vi "Main.vi"() -> ()   [LabVIEW 2015, in "Display.lvlib"]
doc: "This template is based off of the Queued Message Handler design pattern and the Queued Message Handler project template that ships with LabVIEW.\n\nThe main difference is that the queue is private to this module and communication between modules is performed via Broadcast and Request events.\n\nRequest events are wrapped in public API methods and are handled in the Event Handling Loop (EHL) of this VI. Any module can register for Broadcast events sent by this module. The EHL generates messages based on user interface actions.\n\nThe Message Handling Loop (MHL) processes messages generated by the EHL, or by other messages. The messages are string values, so new messages can be added easily to the Message Cases case structure in the MHL. Each message cluster can also provide an optional value for Message Data, which is a variant that can be converted to whatever message-specific data is required.\n_____\nBased on Delacor QMH Project Template 4.2.1.64."
uses:
  Display.lvlib
  <vilib>/Delacor/Delacor QMH/Libraries/Module Admin_class/Delacor_lib_QMH_Module Admin.lvclass
  Module Data--cluster.ctl
  <vilib>/Delacor/Delacor QMH/Libraries/Message Queue_class/Delacor_lib_QMH_Message Queue.lvclass/Delacor_lib_QMH_Message Queue.ctl
  Stop Argument--cluster.ctl
  <vilib>/Delacor/Delacor QMH/Libraries/Module Admin_class/Delacor_lib_QMH_Module Admin.lvclass/Delacor_lib_QMH_Module Admin.ctl
  Update Display Argument--cluster.ctl
  <vilib>/Utility/miscctls.llb/LVPointTypeDef.ctl
  <vilib>/Delacor/Delacor QMH/Libraries/Message Queue_class/Delacor_lib_QMH_Enqueue Message (Single).vi
  <vilib>/Delacor/Delacor QMH/Libraries/Module Admin_class/Delacor_lib_QMH_Get External Launch.vi
  <vilib>/Utility/error.llb/Error Cluster From Error Code.vi
  <vilib>/ErrorRing/Error Ring.xnode
  <vilib>/Delacor/Delacor QMH/Libraries/Message Queue_class/Delacor_lib_QMH_Message Queue.lvclass
panel:
  out "Display":string
  in  "Simulate MHL Error":bool
  in  "Simulate EHL Error":bool
  out "error out":errorcluster
  in  "Module Admin":refnum<class "Delacor_lib_QMH_Module Admin.lvclass">
  out "Status":string
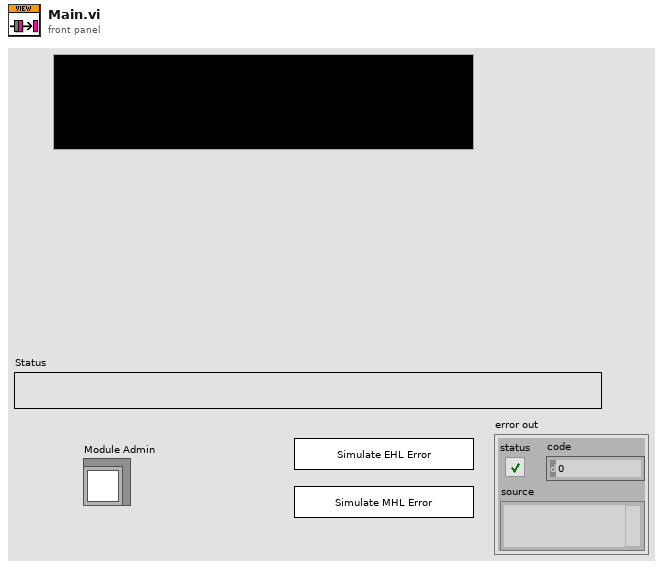
[diagram p1: front panel]
types:
  T1 = typedef "Display.lvlib/Request Events--cluster.ctl" = cluster{"Stop Module":refnum<user-event>, "Show Panel":refnum<user-event>, "Hide Panel":refnum<user-event>, "Get Module Execution Status":refnum<user-event>, "Show Diagram":refnum<user-event>, "Update Display":refnum<user-event>}
  T2 = typedef "Display.lvlib/Module Data--cluster.ctl" = cluster{"Status":string, "Balance (for indication only)":u32}
  T3 = enum32{"invalid lock state", "Not Locked", "Locked (No Password)", "Password-protected"}
  T4 = typedef "Display.lvlib/Stop Argument--cluster.ctl" = cluster{"Origin":string, "Exit via Stop Module Req?":bool, "Wait for Module to stop?":bool}
  T5 = typedef "Display.lvlib/Update Display Argument--cluster.ctl" = cluster{"Message to display":string, "Balance":u32}
  T6 = typedef "LVPointTypeDef.ctl" = cluster{"Horizontal":i16, "Vertical":i16}
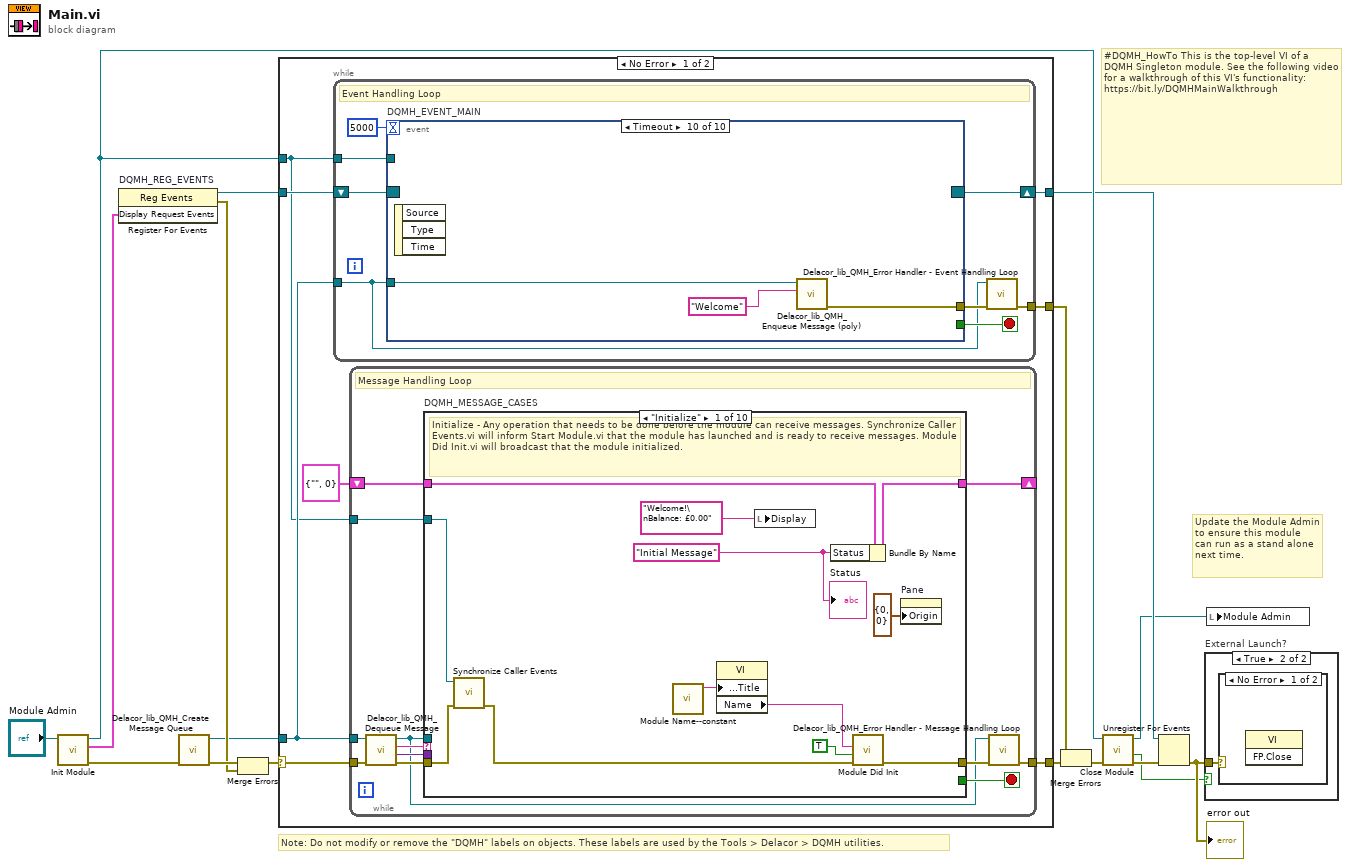
[diagram p0: block diagram]
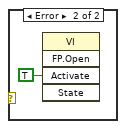
[diagram p3: hidden frame]
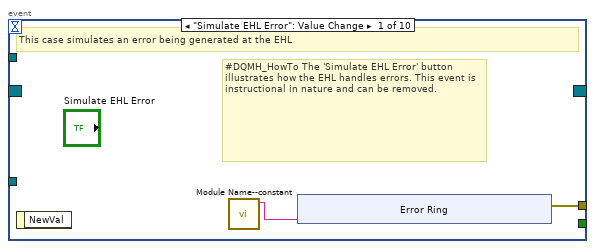
[diagram p4: hidden frame]
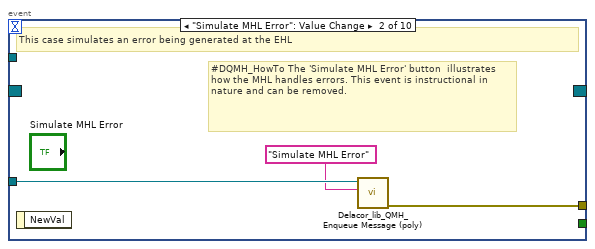
[diagram p5: hidden frame]
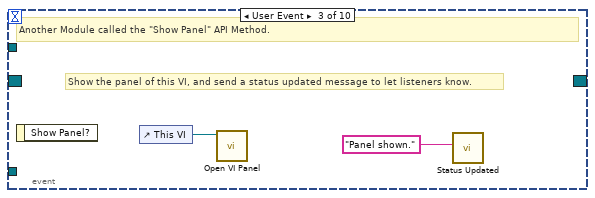
[diagram p6: hidden frame]
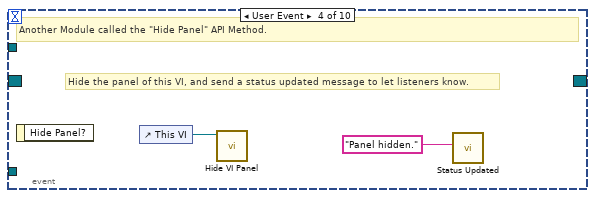
[diagram p7: hidden frame]
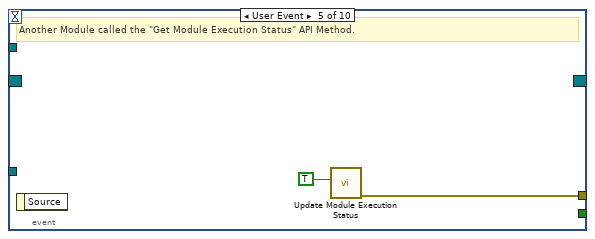
[diagram p8: hidden frame]
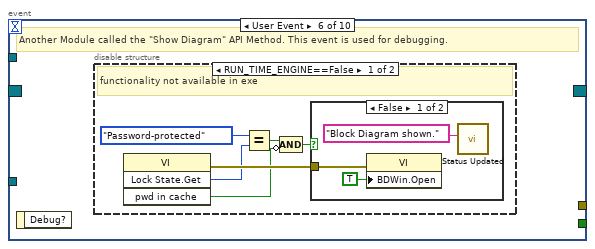
[diagram p9: hidden frame]
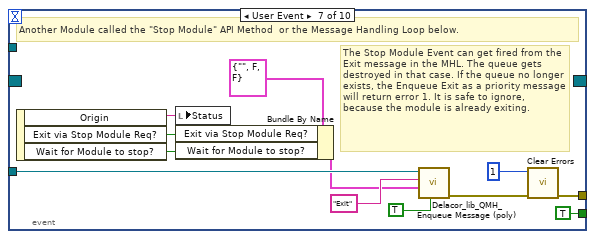
[diagram p12: hidden frame]
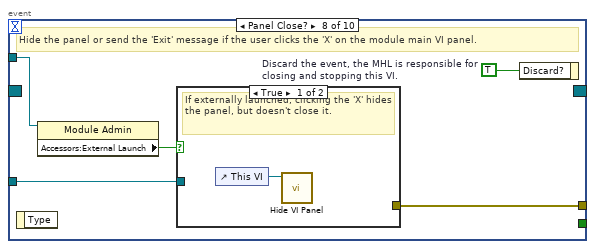
[diagram p13: hidden frame]
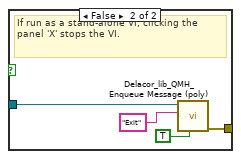
[diagram p14: hidden frame]
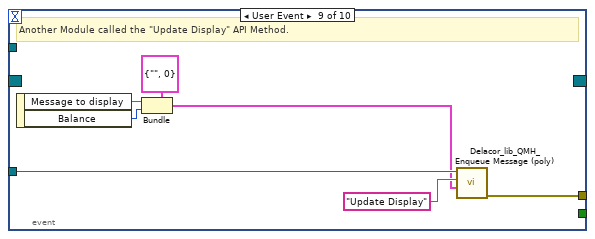
[diagram p15: hidden frame]
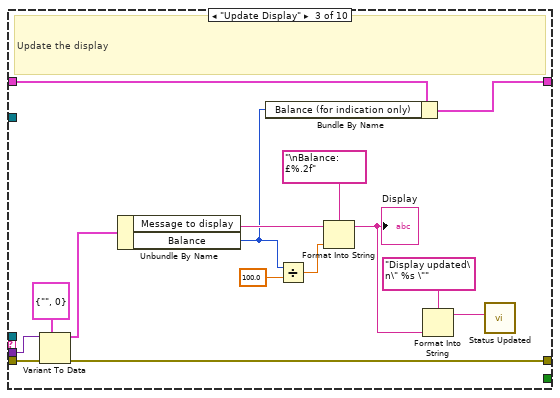
[diagram p17: hidden frame]
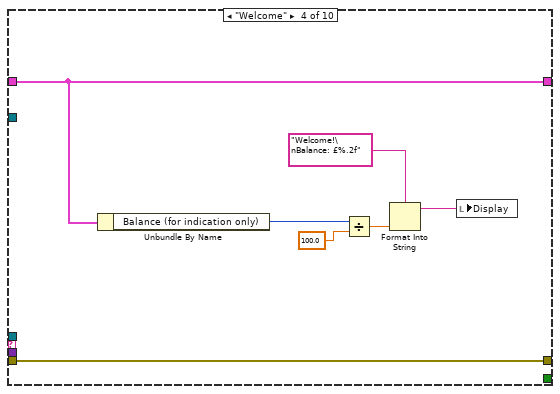
[diagram p18: hidden frame]
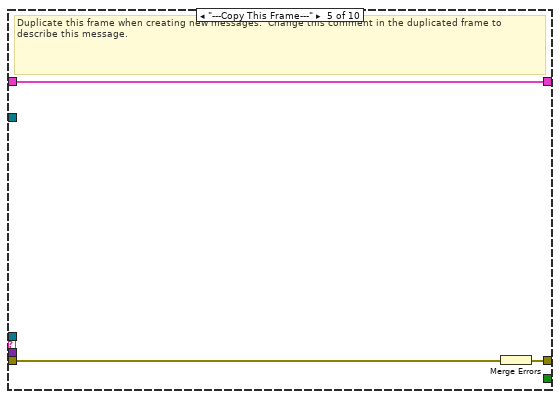
[diagram p19: hidden frame]
diagram:
  # "#DQMH_HowTo This is the top-level VI of a DQMH Singleton module. See the following video for a walkthrough of this VI's functionality: https://bit.ly/DQMHMainWalkthrough"
  # "Note: Do not modify or remove the \"DQMH\" labels on objects. These labels are used by the Tools > Delacor > DQMH utilities."
  # "Update the Module Admin to ensure this module can run as a stand alone next time."
  n1 = call "Init Module.vi"("Singleton Module Admin in"="Module Admin") -> ("error out"=w16:errorcluster, "Display Request Events"=w5:T1, "Singleton Module Admin out"=w8:refnum<class "Delacor_lib_QMH_Module Admin.lvclass">)  [unwired: 8 in]
  n2 = register-events "DQMH_REG_EVENTS"(w5) -> (reference out=w6:refnum<event-registration>, error out=w9:errorcluster)  [unwired: 2 in]
  n3 = call <vilib>:"Delacor_lib_QMH_Create Message Queue.vi"("error in (no error)"=w16) -> ("error out"=w11:errorcluster, "Message Queue"=w4:refnum<class "Delacor_lib_QMH_Message Queue.lvclass">)  [unwired: 9 in]
  n4 = Merge Errors(w11, w9) -> (w10:errorcluster)
  n5 = case shown="No Error" w10 {
    selector: w10 -> [w23 w210]
    tunnel: [w25 w210] -> w17
    tunnel: [w22 w207] -> w7
    tunnel: w6 -> [w20 w207]
    tunnel: w4 -> [w19 _]
    tunnel: [w24 _] -> w14
    tunnel: w8 -> [w18 w203]
    frame No Error {
      n6 = while {
        tunnel: w19 -> [w27]
        shift-right: [w30] -> w22
        shift-left: w20 -> [w31]
        tunnel: [w32] -> w24
        tunnel: w18 -> [w28]
        stop <- w29 stop-if-true
        # "Event Handling Loop"
        n7 = event "DQMH_EVENT_MAIN" shown="[9] Timeout" {
          selector: w31 -> [_ _ _ _ _ _ _ _ _ _]
          dyn-events: [_ _ _ _ _ _ _ _ _ _] -> w30
          timeout: 5000 -> [_ _ _ _ _ _ _ _ _ _]
          tunnel: [_ _ _ _ _ _ TRUE ("Discard?") _ _ _] -> w29
          tunnel: w27 -> [_ w44 _ _ _ _ w68 w75 w89 w90]
          tunnel: [w35 w45 _ _ w51 _ w71 w77 w84 w91] -> w33
          tunnel: w28 -> [_ _ _ _ _ _ _ w74 _ _]
          event "Simulate EHL Error": Value Change {
            # "#DQMH_HowTo The 'Simulate EHL Error' button  illustrates how the EHL handles errors. This event is instructional in nature and can be removed."
            # "This case simulates an error being generated at the EHL"
            n8 = event-data() -> ()  [unwired: 1 in, 1 out]
            n9 = call "Module Name--constant.vi"() -> ("Module Name"=w34:string)  [unwired: 11 in]
            n10 = xnode "Error Ring"("parameter 0"=w34) -> ("error out"=w35:errorcluster)
          }
          event "Simulate MHL Error": Value Change {
            # "#DQMH_HowTo The 'Simulate MHL Error' button  illustrates how the MHL handles errors. This event is instructional in nature and can be removed."
            # "This case simulates an error being generated at the EHL"
            n11 = event-data() -> ()  [unwired: 1 in, 1 out]
            n12 = call-poly <vilib>:"Delacor_lib_QMH_Enqueue Message (poly).vi"("Message"="Simulate MHL Error", "Message Queue in"=w44) -> ("error out"=w45:errorcluster)  [unwired: 8 in, 1 out]
          }
          event User Event {
            # "Show the panel of this VI, and send a status updated message to let listeners know."
            # "Another Module called the \"Show Panel\" API Method."
            n13 = event-data() -> ()  [unwired: 1 in, 1 out]
            n14 = control-ref of="This VI"() -> (w47:refnum<vi>)
            n15 = call "Open VI Panel.vi"("VI"=w47) -> ()  [unwired: 10 in, 1 out]
            n16 = call "Status Updated.vi"("Status"="Panel shown." ("format string")) -> ()  [unwired: 10 in, 1 out]
          }
          event User Event {
            # "Hide the panel of this VI, and send a status updated message to let listeners know."
            # "Another Module called the \"Hide Panel\" API Method."
            n17 = event-data() -> ()  [unwired: 1 in, 1 out]
            n18 = control-ref of="This VI"() -> (w49:refnum<vi>)
            n19 = call "Hide VI Panel.vi"("VI"=w49) -> ()  [unwired: 10 in, 1 out]
            n20 = call "Status Updated.vi"("Status"="Panel hidden." ("format string")) -> ()  [unwired: 10 in, 1 out]
          }
          event User Event {
            # "Another Module called the \"Get Module Execution Status\" API Method."
            n21 = event-data() -> ()  [unwired: 1 in, 1 out]
            n22 = call "Update Module Execution Status.vi"("Running?"=TRUE) -> ("error out"=w51:errorcluster)  [unwired: 10 in]
          }
          event User Event {
            # "Another Module called the \"Show Diagram\" API Method. This event is used for debugging."
            n23 = event-data() -> ()  [unwired: 1 in, 1 out]
            n24 = disable-structure shown="RUN_TIME_ENGINE==False" {
              frame condition #0 (active) {
                # "functionality not available in exe"
                n25 = invoke class="VI" method="Lock State.Get"() -> (error out=w57:errorcluster, "Get Lock State"=w56:T3, "pwd in cache"=w53:bool)  [unwired: 4 in, 1 out]
                n26 = Equal?(x=T3."Password-protected", y=w56) -> (x = y?=w54:bool)
                n27 = Compound Arithmetic op=AND(w54, invert w53) -> (w52:bool)
                n28 = case shown="False" w52 {
                  tunnel: w57 -> [w60 _]
                  frame False {
                    n29 = property class="VI"(error in=w60, "BDWin.Open"=TRUE ("Block Diagram Window:Open")) -> ()  [unwired: 1 in, 2 out]
                    n30 = call "Status Updated.vi"("Status"="Block Diagram shown." ("format string")) -> ()  [unwired: 10 in, 1 out]
                  }
                  frame True {
                    # "Password-protected VI, and the password is not in the cache. Do not show the diagram."
                  }
                }
              }
              frame condition #1 {
              }
            }
          }
          event User Event {
            # "The Stop Module Event can get fired from the Exit message in the MHL. The queue gets destroyed in that case. If the queue no longer exists, the Enqueue Exit as a priority message will return error 1. It is safe to ignore, because the module is already exiting."
            # "Another Module called the \"Stop Module\" API Method  or the Message Handling Loop below."
            n31 = event-data() -> ("Origin"=w67:string, "Exit via Stop Module Req?"=w63:bool, "Wait for Module to stop?"=w62:bool)  [unwired: 1 in]
            n32 = local write "Status"(w67) -> ()
            n33 = Bundle By Name(cluster=T4 {"Origin"="", "Exit via Stop Module Req?"=FALSE, "Wait for Module to stop?"=FALSE} ("Stop Argument"), "Exit via Stop Module Req?"=w63, "Wait for Module to stop?"=w62) -> (w61:T4)
            n34 = call-poly <vilib>:"Delacor_lib_QMH_Enqueue Message (poly).vi"("Priority Message? (F)"=TRUE, "Message Data"=w61, "Message"="Exit", "Message Queue in"=w68) -> ("error out"=w72:errorcluster)  [unwired: 6 in, 1 out]
            n35 = call <vilib>:"Clear Errors.vi"("error in (no error)"=w72, "specific error code to clear (0: all)"=1) -> ("error out"=w71:errorcluster)  [unwired: 4 in, 1 out]
          }
          event Panel Close? {
            w76 = TRUE  # Discard the event, the MHL is responsible for closing and stopping this VI.
            # "Hide the panel or send the 'Exit' message if the user clicks the 'X' on the module main VI panel."
            n36 = event-data() -> ()  [unwired: 1 in, 1 out]
            n37 = property class="Module Admin"(reference=w74) -> ("Accessors:External Launch"=w73:bool)  [unwired: 1 in, 2 out]
            n38 = case shown="True" w73 {
              tunnel: w75 -> [_ w81]
              tunnel: [_ w82] -> w77
              frame True {
                # "If externally launched, clicking the 'X' hides the panel, but doesn't close it."
                n39 = control-ref of="This VI"() -> (w78:refnum<vi>)
                n40 = call "Hide VI Panel.vi"("VI"=w78) -> ()  [unwired: 10 in, 1 out]
              }
              frame False {
                # "If run as a stand-alone VI, clicking the panel 'X' stops the VI."
                n41 = call-poly <vilib>:"Delacor_lib_QMH_Enqueue Message (poly).vi"("Priority Message? (F)"=TRUE, "Message"="Exit", "Message Queue in"=w81) -> ("error out"=w82:errorcluster)  [unwired: 7 in, 1 out]
              }
            }
            n42 = event-data("Discard?"=w76) -> ()  [unwired: 1 in, 1 out]
          }
          event User Event {
            # "Another Module called the \"Update Display\" API Method."
            n43 = event-data() -> ("Message to display"=w85:string, "Balance"=w83:u32)  [unwired: 1 in]
            n44 = Bundle(cluster=T5 {"Message to display"="", "Balance"=0} ("Update Display Argument"), "Message to display"=w85, "Balance"=w83) -> (w86:T5)
            n45 = call-poly <vilib>:"Delacor_lib_QMH_Enqueue Message (poly).vi"("Message Data"=w86, "Message"="Update Display", "Message Queue in"=w89) -> ("error out"=w84:errorcluster)  [unwired: 7 in, 1 out]
          }
          event Timeout {
            n46 = event-data() -> ()  [unwired: 1 in, 3 out]
            n47 = call-poly <vilib>:"Delacor_lib_QMH_Enqueue Message (poly).vi"("Message"="Welcome", "Message Queue in"=w90) -> ("error out"=w91:errorcluster)  [unwired: 8 in, 1 out]
          }
        }
        n48 = call-dynamic "Delacor_lib_QMH_Error Handler - Event Handling Loop.vi"("error in (no error)"=w33, "Message Queue in"=w27) -> ("dup error in"=w32:errorcluster)  [unwired: 8 in, 1 out]
      }
      n49 = while {
        tunnel: w19 -> [w95]
        shift-right: [w99] -> _
        shift-left: T2 {"Status"="", "Balance (for indication only)"=0} ("Data Cluster") -> [w100]
        tunnel: w23 -> [w103]
        tunnel: [w101] -> w25
        tunnel: w18 -> [w93]
        stop <- w98 stop-if-true
        # "Message Handling Loop"
        n50 = call-dynamic "Delacor_lib_QMH_Dequeue Message.vi"("error in (no error)"=w103, "Message Queue in"=w95) -> ("error out"=w102:errorcluster, "Message Data"=w96:variant, "Message"=w97:string, "Message Queue out"=w94:refnum<class "Delacor_lib_QMH_Message Queue.lvclass">)  [unwired: 6 in]
        n51 = case "DQMH_MESSAGE_CASES" shown="\"Initialize\"" w97 {
          selector: w97 -> [_ _ _ _ _ _ _ _ _ w190]
          tunnel: w94 -> [_ _ _ _ _ _ _ w160 w182 _]
          tunnel: w102 -> [w116 w118 w133 w140 w143 w145 w150 w167 w188 w192]
          tunnel: [w114 w118 w132 w140 w142 w145 w149 w163 w185 w193] -> w104
          tunnel: w100 -> [w111 w117 w124 w135 w141 w144 w147 w162 w181 w191]
          tunnel: [w110 w117 w122 w135 w141 w144 w147 w162 w181 w191] -> w99
          tunnel: [_ _ _ _ _ _ _ _ w180 _] -> w98
          tunnel: w96 -> [_ _ w131 _ _ _ _ w161 w179 _]
          tunnel: w93 -> [w112 _ _ _ _ _ _ w159 w174 _]
          frame "Initialize" {
            w107 = "Initial Message" ("Initial Message")
            # "Initialize - Any operation that needs to be done before the module can receive messages. Synchronize Caller Events.vi will inform Start Module.vi that the module has launched and is ready to receive messages. Module Did Init.vi will broadcast that the module initialized."
            n52 = call "Synchronize Caller Events.vi"("error in (no error)"=w116, "Singleton Module Admin in"=w112) -> ("error out"=w115:errorcluster)  [unwired: 8 in, 1 out]
            n53 = call "Module Name--constant.vi"() -> ("Module Name"=w113:string)  [unwired: 11 in]
            n54 = property class="VI"("Front Panel.Title"=w113) -> ("Name"=w105:string)  [unwired: 2 in, 2 out]
            n55 = local write "Display"("Welcome!\nBalance: £0.00" ("Display")) -> ()
            n56 = Bundle By Name(cluster=w111, "Status"=w107) -> (w110:T2)
            n57 = call "Module Did Init.vi"("error in (no error)"=w115, "Initialized?"=TRUE, "Origin"=w105) -> ("error out"=w114:errorcluster)  [unwired: 8 in]
            n58 = property on="Pane" class="Pane"("Origin"=T6 {"Horizontal"=0, "Vertical"=0}) -> ()  [unwired: 2 in, 2 out]
            "Status" <- w107
          }
          frame "--- Module Specific ---" {
            # "Separator -- The following cases handle messages specific to this Module."
          }
          frame "Update Display" {
            # "Update the display"
            n59 = Variant To Data(error in=w133, type=T5 {"Message to display"="", "Balance"=0} ("Update Display Argument"), Variant=w131) -> (data=w129:T5, error out=w132:errorcluster)
            n60 = Unbundle By Name(w129) -> ("Message to display"=w128:string, "Balance"=w123:u32)
            n61 = Bundle By Name(cluster=w124, "Balance (for indication only)"=w123) -> (w122:T2)
            n62 = Divide(x=w123, y=100.0) -> (x/y=w126:dbl)
            n63 = Format Into String(format string="\nBalance: £%.2f", initial string=w128, w126) -> (resulting string=w120:string)  [unwired: 1 in, 1 out]
            "Display" <- w120
            n64 = Format Into String(format string="Display updated\n\" %s \"" ("Status"), w120) -> (resulting string=w119:string)  [unwired: 2 in, 1 out]
            n65 = call "Status Updated.vi"("Status"=w119) -> ()  [unwired: 10 in, 1 out]
          }
          frame "Welcome" {
            n66 = Unbundle By Name(w135) -> ("Balance (for indication only)"=w136:u32)
            n67 = Divide(x=w136, y=100.0) -> (x/y=w138:dbl)
            n68 = Format Into String(format string="Welcome!\nBalance: £%.2f", w138) -> (resulting string=w134:string)  [unwired: 2 in, 1 out]
            n69 = local write "Display"(w134) -> ()
          }
          frame "---Copy This Frame---" {
            # "Duplicate this frame when creating new messages.  Change this comment in the duplicated frame to describe this message."
            n70 = Merge Errors(w143) -> (w142:errorcluster)
          }
          frame "--- Exit and Error Handling---" {
            # "Separator - The following cases handle errors and exit messages."
          }
          frame "Simulate MHL Error" {
            # "#DQMH_HowTo The 'Simulate MHL Error' button  illustrates how the MHL handles errors. This event is instructional in nature and can be removed."
            # "Simulate an error occurring at the MHL"
            n71 = call "Module Name--constant.vi"() -> ("Module Name"=w146:string)  [unwired: 11 in]
            n72 = xnode "Error Ring"("parameter 0"=w146) -> ("error out"=w148:errorcluster)
            n73 = Merge Errors(w150, w148) -> (w149:errorcluster)
          }
          frame "Error" {
            # "#CodeRecommended - If you ever change the name of this \"Error\" message, you'll need to update the name in the Check Loop Error.vi as well."
            # "#CodeRecommended - If the module is running in standalone mode (External Launch = FALSE), this code will pop up an error dialog and call the 'Exit' message if an error occurs. Add more fine-grained error handling here."
            # "Error - Check the error message data and respond accordingly. This message is sent by the \"Error Handler\" VIs at the end of each loop in this application."
            n74 = property class="Module Admin"(reference=w159) -> ("Accessors:External Launch"=w158:bool)  [unwired: 1 in, 2 out]
            n75 = Variant To Data(error in=w167, type=errorcluster {"status"=FALSE, "code"=0, "source"=""} ("error constant"), Variant=w161) -> (data=w168:errorcluster, error out=w165:errorcluster)
            n76 = call "Error Reported.vi"("Error"=w168) -> ()  [unwired: 10 in, 1 out]
            n77 = case shown="False" w158 {
              tunnel: [w173 _] -> w164
              tunnel: w160 -> [w171 _]
              tunnel: w168 -> [w172 _]
              frame False {
                # "If the module is running standalone, then pop up an error dialog and call the \"Exit\" message."
                n78 = call <vilib>:"Simple Error Handler.vi"("error in (no error)"=w172) -> ()  [unwired: 4 in, 5 out]
                n79 = call-poly <vilib>:"Delacor_lib_QMH_Enqueue Message (poly).vi"("Priority Message? (F)"=TRUE, "Message"="Exit", "Message Queue in"=w171) -> ("error out"=w173:errorcluster)  [unwired: 7 in, 1 out]
              }
              frame True {
                # "If the module was launched externally, calling the Error Reported broadcast VI is the only action performed by the \"Error\" message. The module's caller can then process the error appropriately."
              }
            }
            n80 = Merge Errors(w165, w164) -> (w163:errorcluster)
            n81 = local write "error out"(w163) -> ()
          }
          frame "Exit" {
            w178 = 91  # 91: not all Exit messages will have an argument
            w180 = TRUE  # Stop the VI
            # "Release the message queue reference"
            # "#CodeNeeded - Add any required cleanup code here"
            # "Exit - Exit the application."
            n82 = Variant To Data(error in=w188, type=T4 {"Origin"="", "Exit via Stop Module Req?"=FALSE, "Wait for Module to stop?"=FALSE} ("Stop Argument"), Variant=w179) -> (data=w176:T4, error out=w184:errorcluster)
            n83 = call <vilib>:"Clear Errors.vi"("error in (no error)"=w184, "specific error code to clear (0: all)"=w178) -> ("error out"=w187:errorcluster)  [unwired: 4 in, 1 out]
            n84 = control-ref of="This VI"() -> (w175:refnum<vi>)
            n85 = call-dynamic "Delacor_lib_QMH_Release Message Queue.vi"("error in (no error)"=w187, "Message Queue"=w182) -> ("error out"=w186:errorcluster)  [unwired: 9 in]
            n86 = call "Handle Exit.vi"("Stop Argument"=w176, "Admin in"=w174, "VI reference"=w175) -> ("error out"=w183:errorcluster)  [unwired: 7 in, 1 out]
            n87 = Merge Errors(w186, w183) -> (w185:errorcluster)
          }
          frame Default {
            # "'Default' case only runs if there is a message that isn't defined in any of the other cases.  Output a programming error."
            n88 = call "Module Name--constant.vi"() -> ("Module Name"=w189:string)  [unwired: 11 in]
            n89 = xnode "Error Ring"("parameter 0"=w190, "parameter 1"=w189) -> ("error out"=w194:errorcluster)
            n90 = Merge Errors(w192, w194) -> (w193:errorcluster)
          }
        }
        n91 = call-dynamic "Delacor_lib_QMH_Error Handler - Message Handling Loop.vi"("error in (no error)"=w104, "Message Queue in"=w94) -> ("dup error in"=w101:errorcluster)  [unwired: 8 in, 1 out]
      }
    }
    frame Error {
      # "Synchronize Caller Events.vi will inform Start Module.vi that the module has launched and will let the code calling Start Module.vi register for broadcasts and would permit the caller receive the broadcast that an error occurred at launch time."
      n92 = call "Synchronize Caller Events.vi"("Singleton Module Admin in"=w203) -> ("error out"=w208:errorcluster)  [unwired: 9 in, 1 out]
      n93 = call "Module Name--constant.vi"() -> ("Module Name"=w206:string)  [unwired: 11 in]
      n94 = Format Into String(format string="An error occurred during initialization. %s is no longer running.", w206) -> (resulting string=w204:string)  [unwired: 2 in, 1 out]
      n95 = Merge Errors(w210, w208) -> (w209:errorcluster)
      n96 = call "Error Reported.vi"("Additional Information"=w204, "Error"=w209) -> ()  [unwired: 9 in, 1 out]
    }
  }
  n97 = Merge Errors(w14, w17) -> (w13:errorcluster)
  n98 = call "Close Module.vi"("error in (no error)"=w13, "Module Admin in"=w8) -> ("error out"=w15:errorcluster, "External Launch"=w1:bool, "Module Admin out"=w2:refnum<class "Delacor_lib_QMH_Module Admin.lvclass">)  [unwired: 7 in]
  n99 = Unregister For Events(event registration refnum=w7, error in=w15) -> (error out=w12:errorcluster)
  "error out" <- w12
  n100 = case "External Launch?" shown="True" w1 {
    tunnel: w12 -> [_ w211]
    frame False {
    }
    frame True {
      n101 = case shown="No Error" w211 {
        frame No Error {
          n102 = invoke class="VI" method="FP.Close"() -> ()  [unwired: 3 in, 3 out]
        }
        frame Error {
          n103 = invoke class="VI" method="FP.Open"("Activate"=TRUE ("Activate?")) -> ()  [unwired: 4 in, 5 out]
        }
      }
    }
  }
  n104 = local write "Module Admin"(w2) -> ()
